vi "Create Pulse Waveform.vi"(8 "error in (no error)":errorcluster, 11 "RFSoC Driver in":refnum<class "RFSoC Driver.lvclass">) -> (0 "error out":errorcluster, 2 "Array - Numeric":dbl[](array[numeric]), 3 "RFSoC Driver out":refnum<class "RFSoC Driver.lvclass">)   [LabVIEW 2019, in "RFSoC Driver.lvclass"]
uses:
  RFSoC Driver.lvclass
  PulseEcho/PulsedFieldEcho/Create_Pulse/Create_waveform/build_waveform.lvclass
panel:
  out "Waveform Graph":dbl[](graph)
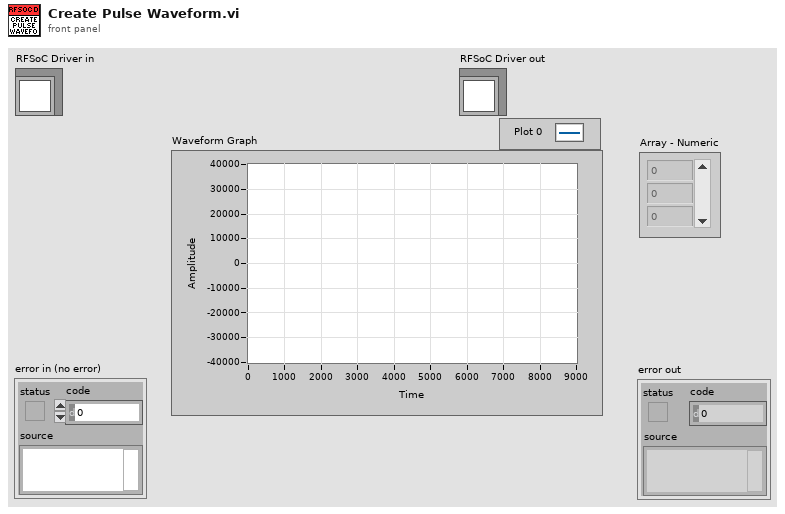
[diagram p1: front panel]
types:
  T1 = typedef "Pulse Parameters.ctl" = cluster{"clock rate":dbl, "Frequency":dbl, "NWaves":i32, "standard deviation":dbl, "Amplitude":dbl, "Mode":enum16{"Sine", "Pulse"}}
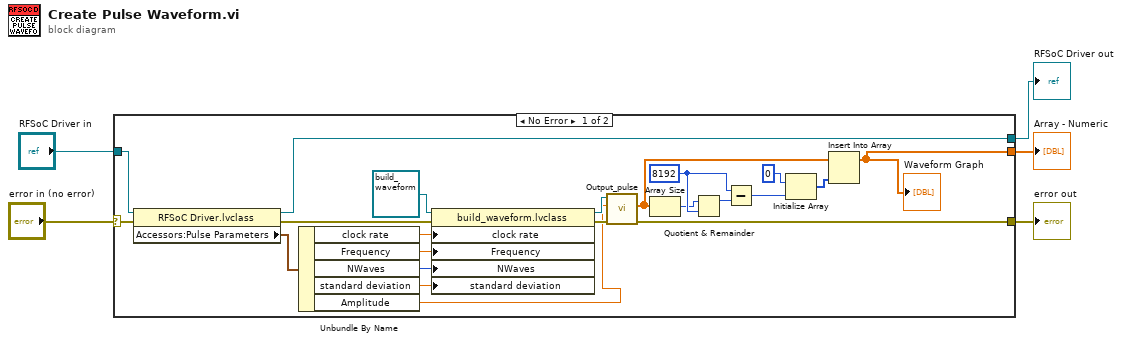
[diagram p0: block diagram]
diagram:
  n1 = case shown="No Error" "error in (no error)" {
    selector: "error in (no error)" -> [w22 w29]
    tunnel: [w12 w29] -> w4
    tunnel: [w8 w28] -> w2
    tunnel: "RFSoC Driver in" -> [w9 w28]
    tunnel: [w11 _] -> w1
    frame No Error {
      w16 = 8192
      n2 = property class="RFSoC Driver.lvclass"(reference=w9, error in=w22) -> (reference out=w8:refnum<class "RFSoC Driver.lvclass">, error out=w10:errorcluster, "Accessors:Pulse Parameters"=w7:T1)
      n3 = Unbundle By Name(w7) -> ("clock rate"=w27:dbl, "Frequency"=w26:dbl, "NWaves"=w25:i32, "standard deviation"=w24:dbl, "Amplitude"=w6:dbl)
      n4 = property class="build_waveform.lvclass"(reference=refnum<class "build_waveform.lvclass"> refnum ("build_waveform.lvclass"), error in=w10, "clock rate"=w27, "Frequency"=w26, "NWaves"=w25, "standard deviation"=w24) -> (reference out=w13:refnum<class "build_waveform.lvclass">, error out=w14:errorcluster)
      n5 = call-dynamic "Output_pulse.vi"("error in (no error)"=w14, "Amplitude"=w6, "build_waveform in"=w13) -> ("error out"=w12:errorcluster, "Array"=w21:dbl[])  [unwired: 6 in, 1 out]
      n6 = Array Size(array=w21) -> (size(s)=w15:i32)
      n7 = Quotient & Remainder(x=w15, y=w16) -> (x-y*floor(x/y)=w17:i32)  [unwired: 1 out]
      n8 = Subtract(x=w16, y=w17) -> (x-y=w20:i32)
      n9 = Initialize Array(i16 0 ("element"), w20) -> (w19:i16[])
      n10 = Insert Into Array(array=w21, new element=w19) -> (w11:dbl[])  [unwired: 1 in]
      "Waveform Graph" <- w11
    }
    frame Error {
    }
  }
  "error out" <- w4
  "RFSoC Driver out" <- w2
  "Array - Numeric" <- w1
